vi "dataset.get_or_create.vi"(8 "error in":errorcluster, 10 "Datascope Name":string, 11 "asset in":refnum<class "asset.lvclass">) -> (0 "error out":errorcluster, 2 "dataset":refnum<class "dataset.lvclass">, 3 "asset out":refnum<class "asset.lvclass">)   [LabVIEW 2020, in "asset.lvclass"]
uses:
  asset.lvclass
  Nominal Client/datasources/dataset/dataset.lvclass
  asset.lvclass/asset.ctl
  Nominal Client/Nominal Client.lvclass
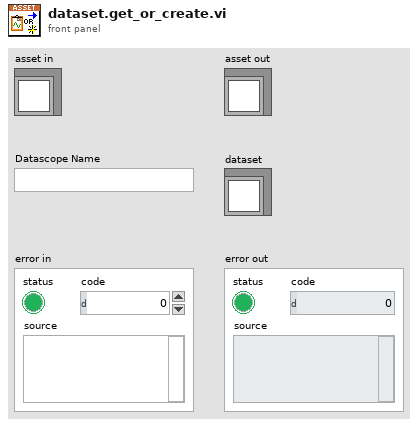
[diagram p1: front panel]
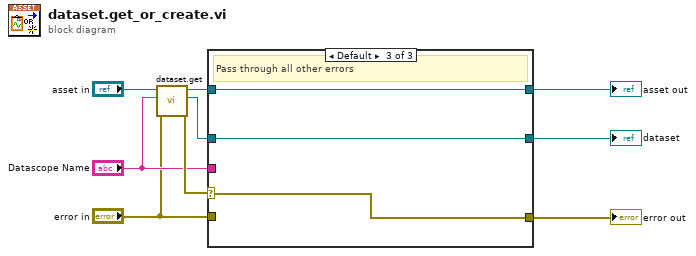
[diagram p0: block diagram]
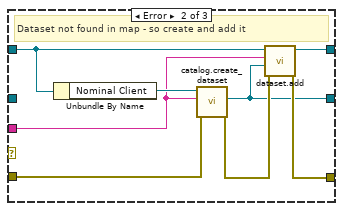
[diagram p3: hidden frame]
diagram:
  n1 = call "dataset.get.vi"("error in"="error in", "Datascope Name"="Datascope Name", "asset in"="asset in") -> ("error out"=w5:errorcluster, "dataset"=w6:refnum<class "dataset.lvclass">, "asset out"=w8:refnum<class "asset.lvclass">)  [unwired: 6 in]
  n2 = case shown="Default" w5 {
    selector: w5 -> [w10 _ w21]
    tunnel: w8 -> [w12 w19 w23]
    tunnel: [w12 w18 w23] -> w7
    tunnel: w6 -> [w11 _ w22]
    tunnel: [w11 w14 w22] -> w4
    tunnel: [w10 w15 w21] -> w3
    tunnel: "Datascope Name" -> [_ w17 _]
    tunnel: "error in" -> [_ w13 _]
    frame No Error {
      # "Dataset found"
    }
    frame Error {
      # "Dataset not found in map - so create and add it"
      n3 = Unbundle By Name(w19) -> ("Nominal Client"=w20:refnum<class "Nominal Client.lvclass">)
      n4 = call "catalog.create_dataset.vi"("error in"=w13, "name"=w17, "Nominal Client in"=w20) -> ("error out"=w16:errorcluster, "Dataset"=w14:refnum<class "dataset.lvclass">)  [unwired: 6 in, 1 out]
      n5 = call "dataset.add.vi"("error in"=w16, "dataset"=w14, "Datascope Name"=w17, "asset in"=w19) -> ("error out"=w15:errorcluster, "asset out"=w18:refnum<class "asset.lvclass">)  [unwired: 6 in]
    }
    frame Default {
      # "Pass through all other errors"
    }
  }
  "asset out" <- w7
  "error out" <- w3
  "dataset" <- w4
